vi "Custom Device Section.vi"(8 "error in (no error)":errorcluster, 11 "Node Ptr":u64) -> (0 "error out":errorcluster)   [LabVIEW 2013, in "Custom Device.lvlib"]
uses:
  Custom Device.lvlib
  System Explorer Framework/Section Divider.ctl
  Communication Layer/FGVActions.ctl
  Shared/NIVS_Shared.lvlib
  Communication Layer/Communication.lvlib
  Shared/System Storage/Tree Storage/Tree Storage.lvlib
  System Explorer Framework/System Explorer Framework.lvlib
panel:
  in  "Header":T1={"Section Name"="Custom Device Section Specification"}
  out "Name":string
  in  "Description":string
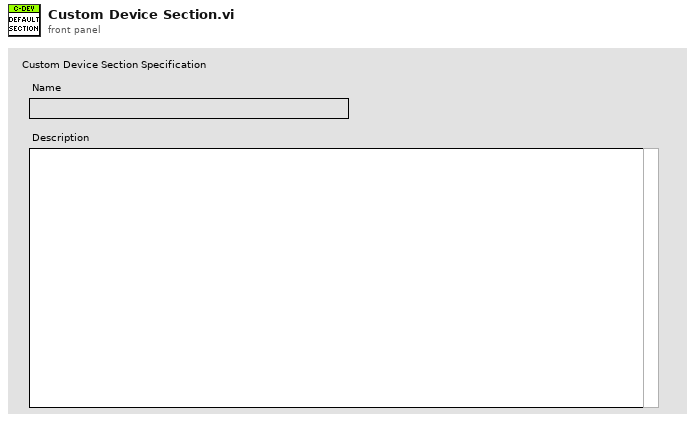
[diagram p1: front panel]
types:
  T1 = typedef "System Explorer Framework.lvlib/Section Divider.ctl" = cluster{"Section Name":string}
  T2 = typedef "Communication.lvlib/FGVActions.ctl" = enum16{"Generate Event", "Get Event Ref", "Create Event", "Destroy"}
  T3 = typedef "NIVS_DataStorage.lvlib/BaseNodeType.ctl" = refnum<k24>
  T4 = typedef "Communication.lvlib/General Communication Action.ctl" = enum16{"Event structure", "Unsaved", "Release FP Cursor", "Set FP Cursor Busy", "Refresh (Flood)", "Refresh (Add)", "Refresh (Add no highlight)", "Refresh (Repopulate certain node)", "Refresh (Update)", "Refresh (Delete)", "Refresh (Delete no highlight)", "Refresh (Rename)", "Refresh (Move)", "Refresh (Move no highlight)", "Refresh (no highlight)", "Refresh (CD)", "Refresh (single nodes)", "Stop", "GW_WD: Save", "GW_WD: Add Items", "GW_WD: Add Items (no highlight)", "GW_WD: Add Item (CD)", "GW_WD: Update Items", "GW_WD: Delete Item", "GW_WD: Delete Item (no highlight)", "GW_WD: Force Delete Item (no highlight)", "GW_WD: Force Delete Item (no highlight - requested item only)", "GW_WD: Force Delete Item (no highlight - requested item only / Skip Action VI)", "GW_WD: Rename Item", "GW_WD: Move Item", "GW_WD: Repopulate Node", "GW_WD: Load Data from Disk", "GW_WD: Import Data", "GW_WD: New", "GW_WD: Action on Save", "GW_WD: Action on System Shutdown", "GW_WD: Ask save SDF", "GW_WD: Add Revision", "GW_WD: Filter Stop", "GW_WD: Open", "GW_WD: Action on Load", "GW_WD: Save as...", "GW_WD: Deploy", "GW_WD: Close System Explorer", "GW_WD: Current page commit changes", "GW_WD: Current page shutdown", "GW_WD: Add Rev History", "GW_WD: Wait on Action Load", "GW_WD: Signalize Load is Done", "GW_WD: Open File", "GW_WD: Wait on Action Save", "GW_WD: Wait on Action Delete", "GW_WD: Signalize Action Save is Done", "GW_WD: Signalize Action Delete is Done", "GW_WD: Hide Progress Dialog", "GW_WD: Show Progress Dialog", "Delete Cancelled", "GW_WD: Relaunch Page", "GW_WD: Add Item (CD no highlight)", "GW_WD: Activate Progress Window", "GW_WD: Close Progress Window", "GW_WD: Buffering Enabled", "GW_WD: Commit Changes", "GW_WD: Delete Item (notification)", "GW_WD: Force Delete Item (no highlight - notification)", "Page: Send Button ID", "GW_WD: Copy", "GW_WD: Cut", "GW_WD: Paste", "GW_WD: Warning", "GW_WD: Wait on Action Paste", "GW_WD: Signalize Action Paste is Done", "GW_WD: Items Added (highlight)", "GW_WD: Items Added (no highlight)", "GW_WD: Items Added (no highlight / skip action VI)", "GW_WD: Items Added (repopulate certain node)", "GW_WD: Launch Busy Dialog Data Storage", "GW_WD: Stop Busy Dialog Data Storage", "Enable Dynamic Button", "Disable Dynamic Button", "GW_WD: Items Deleted", "GW_WD: Items Deleted (no highlight)", "Insert VI Into SubPanel", "Highlight item", "Update Error Count"}
  T5 = typedef "Communication.lvlib/Listener.ctl" = enum16{"ALL", "System Explorer", "SubPanel VI", "Dialog VI", "Action VI", "GW_WD", "Individual Listener"}
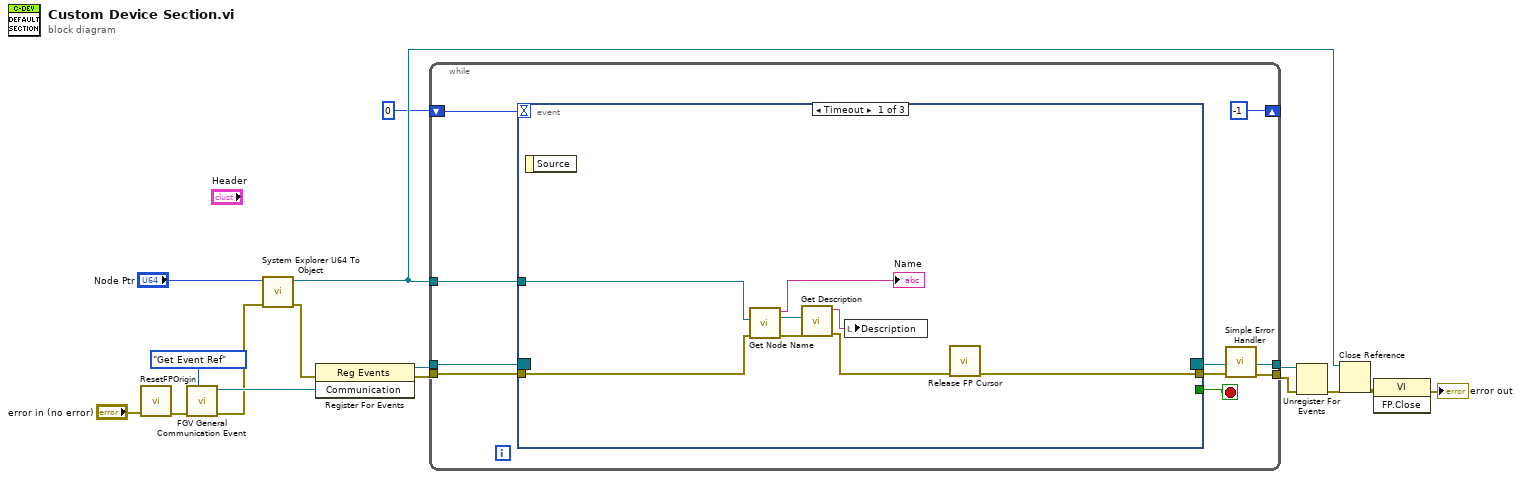
[diagram p0: block diagram]
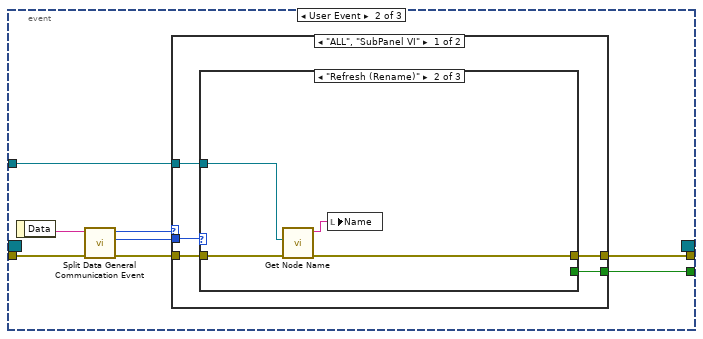
[diagram p2: hidden frame]
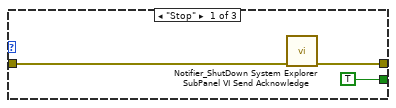
[diagram p3: hidden frame]
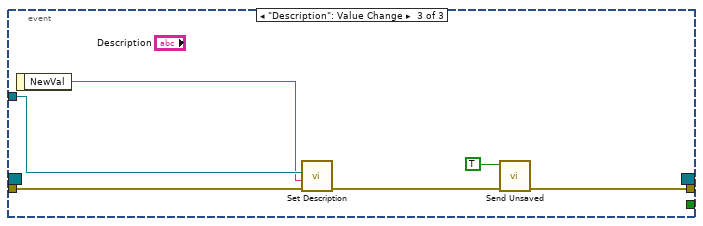
[diagram p6: hidden frame]
diagram:
  n1 = call "ResetFPOrigin.vi"("error in (no error)"="error in (no error)") -> ("error out"=w8:errorcluster)  [unwired: 1 in, 9 out]
  n2 = call "FGV General Communication Event.vi"("Action"=FGVActions."Get Event Ref", "error in (no error)"=w8) -> ("error out"=w3:errorcluster, "Communication"=w12:refnum<user-event>)  [unwired: 1 in, 7 out]
  n3 = call "System Explorer U64 To Object.vi"("error in (no error)"=w3, "Node Ptr"="Node Ptr") -> ("error out"=w2:errorcluster, "NodeObject"=w4:T3)  [unwired: 7 in, 1 out]
  n4 = register-events(error in=w2, w12) -> (reference out=w10:refnum<event-registration>, error out=w11:errorcluster)  [unwired: 1 in]
  n5 = while {
    tunnel: [w25] -> w16
    tunnel: [w24] -> w15
    tunnel: w11 -> [w23]
    tunnel: w10 -> [w22]
    tunnel: w4 -> [w19]
    shift-right: [-1] -> _
    shift-left: 0 -> [w18]
    stop <- w20 stop-if-true
    n6 = event shown="[0] Timeout" {
      selector: w22 -> [_ _ _]
      dyn-events: [_ _ _] -> w25
      timeout: w18 -> [_ _ _]
      tunnel: w23 -> [w33 w39 w59]
      tunnel: [_ w41 _] -> w20
      tunnel: [w32 w40 w61] -> w21
      tunnel: w19 -> [w30 w34 w57]
      event Timeout {
        n7 = event-data() -> ()  [unwired: 2 out]
        n8 = call "Get Node Name.vi"("error in (no error)"=w33, "BaseNdType"=w30) -> ("error out"=w29:errorcluster, "BaseNdType"=w28:T3, "Node Name"=→"Name":string)  [unwired: 7 out]
        n9 = call "Get Description.vi"("error in (no error)"=w29, "BaseNdType in"=w28) -> ("error out"=w26:errorcluster, "Description"=w27:string)  [unwired: 6 in, 2 out]
        n10 = local write "Description"(w27) -> ()
        n11 = call "Release FP Cursor.vi"("error in (no error)"=w26) -> ("error out"=w32:errorcluster)  [unwired: 10 out]
      }
      event User Event {
        n12 = event-data() -> ("Data"=w38:string)  [unwired: 1 out]
        n13 = call "Split Data General Communication Event.vi"("error in"=w39, "Data"=w38) -> ("error out"=w37:errorcluster, "Action"=w35:T4, "Listener"=w36:T5)  [unwired: 7 out]
        n14 = case shown="\"ALL\", \"SubPanel VI\"" w36 {
          tunnel: w37 -> [w45 w55]
          tunnel: w35 -> [w46 _]
          tunnel: [w44 _] -> w41
          tunnel: [w43 w55] -> w40
          tunnel: w34 -> [w42 _]
          frame "ALL", "SubPanel VI" {
            n15 = case shown="\"Refresh (Rename)\"" w46 {
              tunnel: w45 -> [w47 w53 w54]
              tunnel: [w49 w51 w54] -> w43
              tunnel: [TRUE _ _] -> w44
              tunnel: w42 -> [_ w50 _]
              frame "Stop" {
                n16 = call "Notifier_ShutDown System Explorer SubPanel VI Send Acknowledge.vi"("error in (no error)"=w47) -> ("error out"=w49:errorcluster)  [unwired: 1 in, 9 out]
              }
              frame "Refresh (Rename)" {
                n17 = call "Get Node Name.vi"("error in (no error)"=w53, "BaseNdType"=w50) -> ("error out"=w51:errorcluster, "Node Name"=w52:string)  [unwired: 8 out]
                n18 = local write "Name"(w52) -> ()
              }
              frame Default {
              }
            }
          }
          frame Default {
          }
        }
      }
      event "Description": Value Change {
        n19 = event-data() -> ("NewVal"=w56:string)  [unwired: 1 out]
        n20 = call "Set Description.vi"("error in (no error)"=w59, "Description"=w56, "BaseNdType in"=w57) -> ("error out"=w58:errorcluster)  [unwired: 6 in, 2 out]
        n21 = call "Send Unsaved.vi"("error in (no error)"=w58, "Send unsaved? (T)"=TRUE) -> ("error out"=w61:errorcluster)  [unwired: 9 out]
      }
    }
    n22 = call <vilib>:"Simple Error Handler.vi"("error in (no error)"=w21) -> ("error out"=w24:errorcluster)  [unwired: 1 in, 7 out]
  }
  n23 = Unregister For Events(event registration refnum=w16, error in=w15) -> (error out=w6:errorcluster)
  n24 = Close Reference(reference=w4, error in (no error)=w6) -> (error out=w5:errorcluster)
  n25 = invoke class="VI" method="FP.Close"(error in=w5) -> (error out=→"error out":errorcluster)  [unwired: 2 in, 2 out]
